vi "I32toByteArray.vi"(8 "error in (no error)":errorcluster, 11 "I32":i32) -> (0 "error out":errorcluster, 3 "LittleEndianByteArray":u8[](array[numeric]))   [LabVIEW 2013, in "BSON.lvlib"]
uses:
  BSON.lvlib
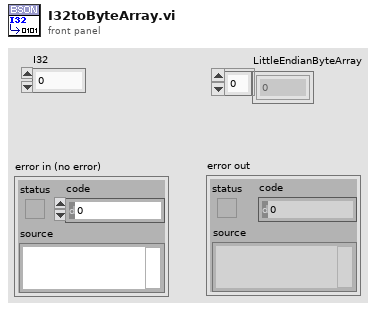
[diagram p1: front panel]
types:
  T1 = enum16{"big-endian, network order", "native, host order", "little-endian"}
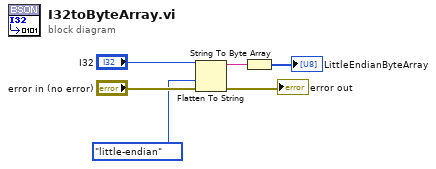
[diagram p0: block diagram]
diagram:
  n1 = Flatten To String(anything="I32", byte order (0:big-endian, network order)=T1."little-endian", error in (no error)="error in (no error)") -> (data string=w3:string, error out=→"error out":errorcluster)  [unwired: 1 in, 1 out]
  n2 = String To Byte Array(string=w3) -> (unsigned byte array=→"LittleEndianByteArray":u8[])
